vi "remove_files.vi"(1 "Hora de borrado":string) -> ()   [LabVIEW 2015]
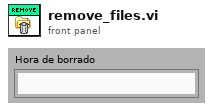
[diagram p1: front panel]
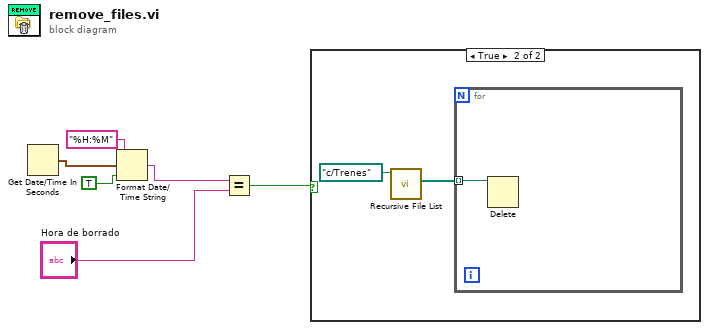
[diagram p0: block diagram]
diagram:
  n1 = Get Date/Time In Seconds() -> (seconds since 1Jan1904=w4:timestamp)
  n2 = Format Date/Time String(time format string (%c)="%H:%M", seconds (now)=w4, UTC format=TRUE) -> (date/time string=w3:string)
  n3 = Equal?(x=w3, y="Hora de borrado") -> (x = y?=w1:bool)
  n4 = case shown="True" w1 {
    frame False {
    }
    frame True {
      n5 = call <vilib>:"Recursive File List.vi"("Folder Path"=path "c:/Trenes") -> ("All Files in Dir"=w7:path[])  [unwired: 6 in, 4 out]
      n6 = for {
        tunnel: w7 -> [w9] mode=indexing
        n7 = Delete(path (use dialog)=w9) -> ()  [unwired: 4 in, 3 out]
      }
    }
  }
